vi "FILTER_BOX_30.vi"(10 "Input":dbl) -> (2 "Filtered_Value":dbl)   [LabVIEW 2019]
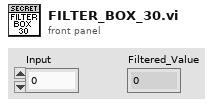
[diagram p1: front panel]
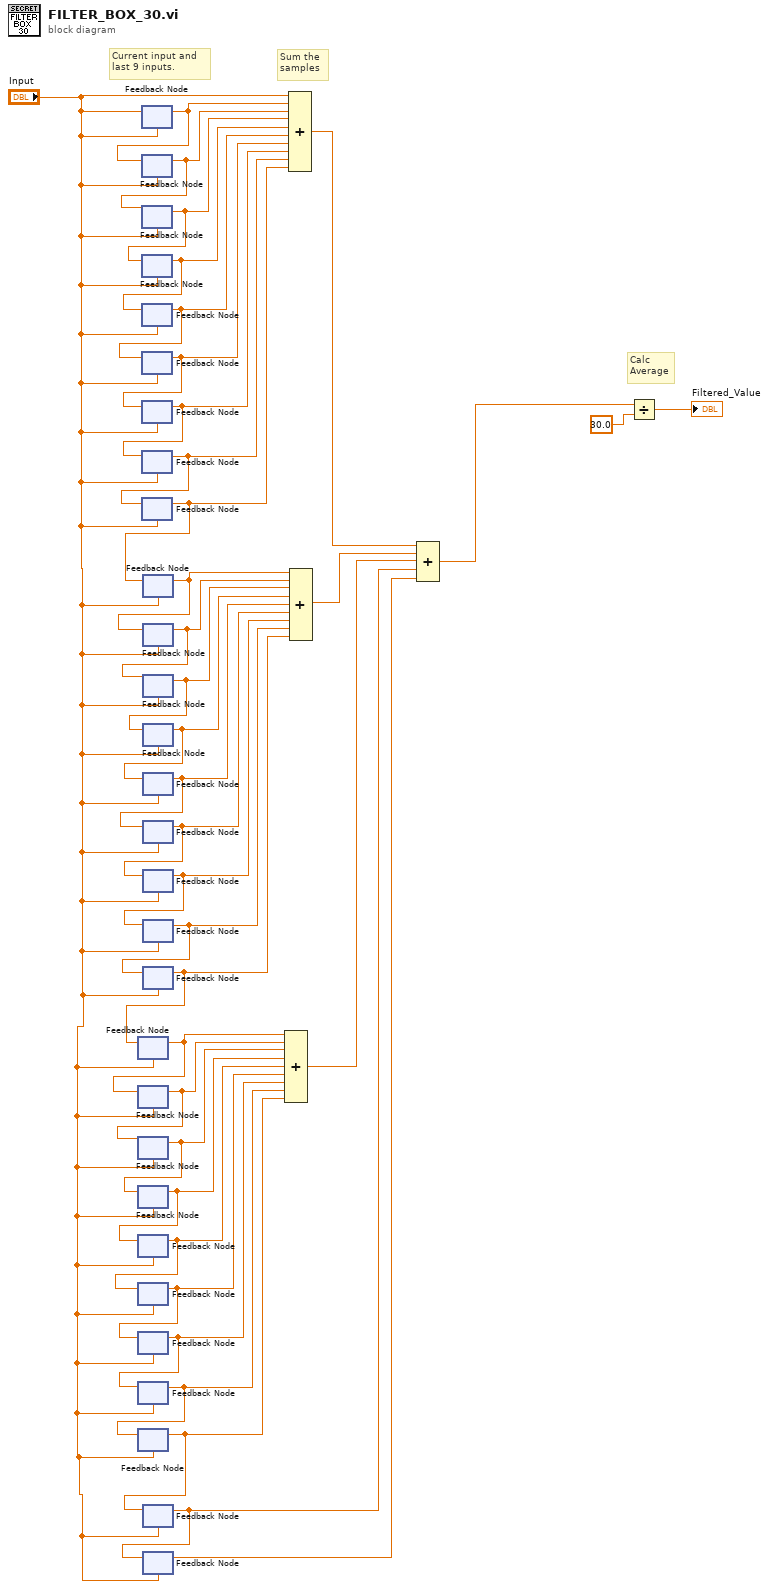
[diagram p0: block diagram]
diagram:
  # "Current input and \nlast 9 inputs."
  # "Calc\nAverage"
  # "Sum the \nsamples"
  n1 = feedback #1("Input") -> (w18:dbl)
  n2 = feedback #2("Input") -> (w17:dbl)
  n3 = feedback-in #2(w18) -> ()
  n4 = feedback #3("Input") -> (w16:dbl)
  n5 = feedback-in #3(w17) -> ()
  n6 = feedback #4("Input") -> (w15:dbl)
  n7 = feedback-in #4(w16) -> ()
  n8 = feedback #5("Input") -> (w14:dbl)
  n9 = feedback-in #5(w15) -> ()
  n10 = feedback #6("Input") -> (w13:dbl)
  n11 = feedback-in #6(w14) -> ()
  n12 = feedback #7("Input") -> (w12:dbl)
  n13 = feedback-in #7(w13) -> ()
  n14 = feedback #8("Input") -> (w11:dbl)
  n15 = feedback-in #8(w12) -> ()
  n16 = feedback #9("Input") -> (w8:dbl)
  n17 = feedback-in #9(w11) -> ()
  n18 = feedback-in #10("Input") -> ()
  n19 = feedback #10("Input") -> (w36:dbl)
  n20 = feedback #11("Input") -> (w35:dbl)
  n21 = feedback-in #11(w36) -> ()
  n22 = feedback #12("Input") -> (w34:dbl)
  n23 = feedback-in #12(w35) -> ()
  n24 = feedback #13("Input") -> (w33:dbl)
  n25 = feedback-in #13(w34) -> ()
  n26 = feedback #14("Input") -> (w32:dbl)
  n27 = feedback-in #14(w33) -> ()
  n28 = feedback #15("Input") -> (w31:dbl)
  n29 = feedback-in #15(w32) -> ()
  n30 = feedback #16("Input") -> (w30:dbl)
  n31 = feedback-in #16(w31) -> ()
  n32 = feedback #17("Input") -> (w29:dbl)
  n33 = feedback-in #17(w30) -> ()
  n34 = feedback #18("Input") -> (w10:dbl)
  n35 = feedback-in #18(w29) -> ()
  n36 = feedback #19("Input") -> (w26:dbl)
  n37 = feedback-in #19(w10) -> ()
  n38 = feedback #20("Input") -> (w25:dbl)
  n39 = feedback-in #20(w26) -> ()
  n40 = feedback #21("Input") -> (w24:dbl)
  n41 = feedback-in #21(w25) -> ()
  n42 = feedback #22("Input") -> (w23:dbl)
  n43 = feedback-in #22(w24) -> ()
  n44 = feedback #23("Input") -> (w22:dbl)
  n45 = feedback-in #23(w23) -> ()
  n46 = feedback #24("Input") -> (w21:dbl)
  n47 = feedback-in #24(w22) -> ()
  n48 = feedback #25("Input") -> (w20:dbl)
  n49 = feedback-in #25(w21) -> ()
  n50 = feedback #26("Input") -> (w19:dbl)
  n51 = feedback-in #26(w20) -> ()
  n52 = feedback #27("Input") -> (w9:dbl)
  n53 = feedback-in #1(w9) -> ()
  n54 = feedback-in #27(w19) -> ()
  n55 = feedback #28("Input") -> (w3:dbl)
  n56 = feedback-in #28(w8) -> ()
  n57 = feedback #29("Input") -> (w2:dbl)
  n58 = feedback-in #29(w3) -> ()
  n59 = Compound Arithmetic op=ADD(w18, w17, w16, w15, w14, w13, w12, w11, w8) -> (w4:dbl)
  n60 = Compound Arithmetic op=ADD("Input", w36, w35, w34, w33, w32, w31, w30, w29, w10) -> (w6:dbl)
  n61 = Compound Arithmetic op=ADD(w26, w25, w24, w23, w22, w21, w20, w19, w9) -> (w5:dbl)
  n62 = Compound Arithmetic op=ADD(w6, w5, w4, w3, w2) -> (w1:dbl)
  n63 = Divide(x=w1, y=30.0) -> (x/y=→"Filtered_Value":dbl)
